vi "Main Monitor Loop.vi"(8 "error in (no error)":errorcluster, 11 "main ref":T1) -> (0 "error out":errorcluster)   [LabVIEW 2025]
uses:
  controls/LAB-IQ UI Data.ctl
  Traction Loop/Traction Receipe Enum.ctl
  <vilib>/Utility/error.llb/Trim Whitespace One-Sided.vi
panel:
  out "TDMS CLOSE":bool
  out "tdms file out":refnum<k34>
  out "File Create Temp":bool
  out "error out 2":errorcluster
  out "Test Stop Temp":bool
  out "DepthZ":dbl
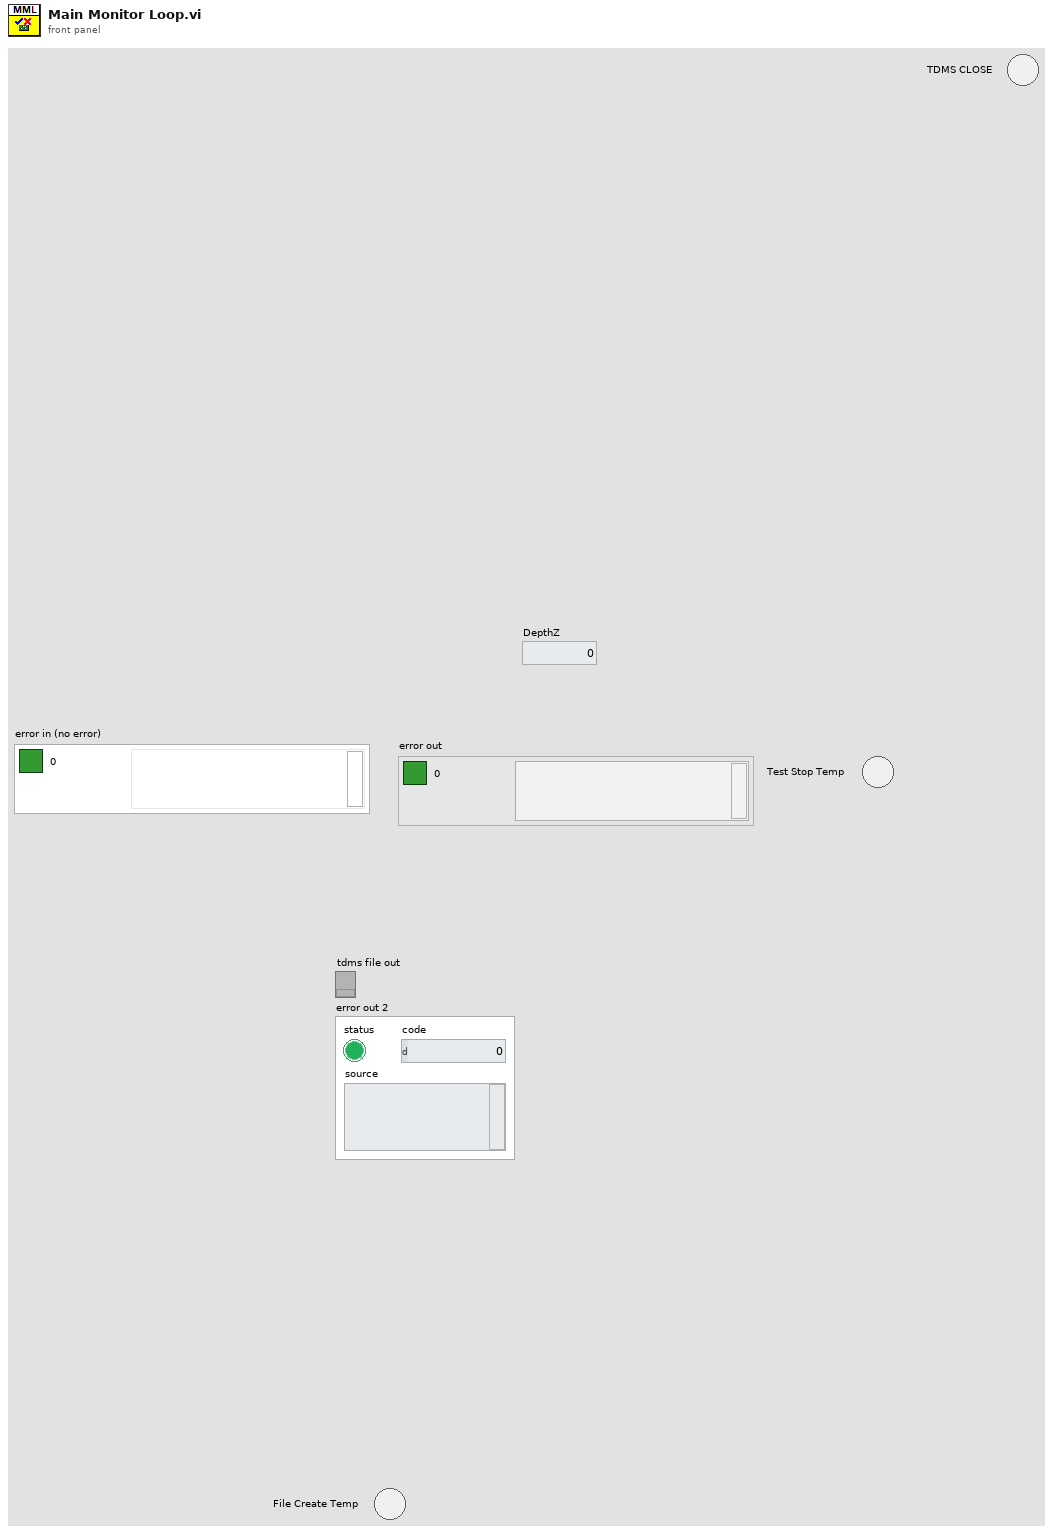
[diagram p1: front panel]
types:
  T1 = typedef "LAB-IQ UI Data.ctl" = cluster{"Main Home Screen":cluster{"GUI":refnum<vi>, "Platform Settings":refnum<vi>, "Configure":refnum<vi>, "Home":refnum<vi>, "EXIT":refnum<vi>, "service 2":refnum<vi>, "MainPage":refnum<vi>, "Analysis":refnum<vi>}, "Platform Settings":cluster{"mm/s  Surge":refnum<vi>, "Drive Error":refnum<vi>, "Disable Axis Jog Soft Limits":refnum<vi>, "mm/s  Sway":refnum<vi>, "Sway and Surge COM Status":refnum<vi>, "Heave COM Status":refnum<vi>, "Enable Platform":refnum<vi>, "Surge Forward Main":refnum<vi>, "Sway Right Main":refnum<vi>, "Sway Left Main":refnum<vi>, "Heave Down Main":refnum<vi>, "Heave Up main":refnum<vi>, "mm/s Heave":refnum<vi>, "mm/sec":refnum<vi>, "mm":refnum<vi>, "Surge Backward Main":refnum<vi>}, "Analysis Screen":cluster{"Analysis Home":refnum<vi>, "Surface Analysis":refnum<vi>, "Imaging":refnum<vi>, "Image Analysis":refnum<vi>, "Post Analysis":refnum<vi>}, "Config Screen":cluster{"Select Load Head":refnum<vi>, "Notes :":refnum<vi>, "FILE":refnum<vi>, "Sample ID :":refnum<vi>, "Operator ID :":refnum<vi>, "Operator Name :":refnum<vi>, "Auto":refnum<vi>}, "Motion Module":cluster{"zNL":refnum<vi>, "NL disp":refnum<vi>, "Rotary Tab":refnum<vi>, "Motion Direction:  3":refnum<vi>, "E.Velocity 2":refnum<vi>, "e.v/ssr 2":refnum<vi>, "Enter Fixed E.Velocity 2":refnum<vi>, "Enter Final SRR 2":refnum<vi>, "Enter initial SRR 2":refnum<vi>, "Enter Fixed SRR 2":refnum<vi>, "Enter the Final E.Velocity (m/s) 2":refnum<vi>, "Enter initial E.Velocity (m/s) 2":refnum<vi>, "Final Speed (RPM) 3":refnum<vi>, "Initial Speed (RPM) 2":refnum<vi>, "Enter the Final Velocity (m/s) 3":refnum<vi>, "Enter initial Velocity (m/s)  3":refnum<vi>, "Ramp Up 2":refnum<vi>, "TEST SELECTION":refnum<vi>, "SPEED SELECTION : ":refnum<vi>, "Angular Oscillation Set":refnum<vi>, "Traction":refnum<vi>, "Step Speed":refnum<vi>, "StepTable For Load-Speed":refnum<vi>, "StepTable For Speed":refnum<vi>, "Surge Forward MM":refnum<vi>, "Surge Backward MM":refnum<vi>, "M3 Image":refnum<vi>, "String 39":refnum<vi>, "Sway Left MM":refnum<vi>, "Sway Right MM":refnum<vi>, "Disable Axis Jog Soft Limits":refnum<vi>, "mm":refnum<vi>, "Heave Down MM":refnum<vi>, "Heave Up MM":refnum<vi>, "Wear Track Diameter (mm)":refnum<vi>, "Set WTD":refnum<vi>, "HomeScratch":refnum<vi>, "HomeRot":refnum<vi>, "PlaceModule":refnum<vi>, "Enter the Angle (Deg)":refnum<vi>, "Enter the Frequency (Hz)":refnum<vi>, "Motion Mode:":refnum<vi>, "LR Sway":refnum<vi>, "Rot Hor":refnum<vi>, "Scratch":refnum<vi>, "LR Cam":refnum<vi>, "MMBack":refnum<vi>, "MMNext":refnum<vi>, "Rot Ver":refnum<vi>, "Rotary Module Selection":refnum<vi>, "calculate rotary":refnum<vi>, "SPEED SELECTION : rotary":refnum<vi>, "Import 2":refnum<vi>, "Save 2":refnum<vi>, "File Path :  2":refnum<vi>, "String 45":refnum<vi>, "StepTable For Speed 3":refnum<vi>, "Enter the Speed(mm/sec)":refnum<vi>, "Enter the Speed(RPM)":refnum<vi>, "Enter Scratch Speed (mm/s):":refnum<vi>, "SwaySpeed Set":refnum<vi>, "Scartch Offset":refnum<vi>, "Motion type:":refnum<vi>, "HomeScratch 2":refnum<vi>, "Enter Scratch length (mm):":refnum<vi>, "Wear Track Diameter":refnum<vi>, "Rotary Speed Exced":refnum<vi>, "Scratch Mode":refnum<vi>, "No of Scratch":refnum<vi>}, "Environmental control":cluster{"Humidity  Status  3":refnum<vi>, "Low Temp  Status  2":refnum<vi>, "TK4 status 2":refnum<vi>, "Stage Temperature":refnum<vi>, "Sample Temperature":refnum<vi>, "Humidity (Amb)":refnum<vi>, "Clear List":refnum<vi>, "Add to list":refnum<vi>, "Wear":refnum<vi>, "Vibration":refnum<vi>, "Humidity (Chamber)":refnum<vi>, "Temperature (Chamber)":refnum<vi>, "ECR ":refnum<vi>, "Temperature (Amb)":refnum<vi>, "Microphone":refnum<vi>, "Acoustic Emission 3":refnum<vi>, "SNext":refnum<vi>, "APBack":refnum<vi>, "Enter the Temperature (°C):":refnum<vi>, "Enter the Stage \nTemperature (°C):":refnum<vi>, "Enter the Humidity (%Rh):":refnum<vi>, "Low Temp":refnum<vi>, "High Temp":refnum<vi>, "Humidity":refnum<vi>, "Sensors Picked":refnum<vi>}, "About Screen":cluster{"Password":refnum<vi>, "Home Service":refnum<vi>, "Advanced Setting":refnum<vi>, "About Tab":refnum<vi>, "ECR Port:":refnum<vi>, "Ramp Port:":refnum<vi>, "Installation/Replacement completed":refnum<vi>, "Loahead":refnum<vi>, "Heave and Surge COM Port:":refnum<vi>, "Sway COM Port:":refnum<vi>, "Temp Modbus:":refnum<vi>, "Humidity Port:":refnum<vi>, "Edit Gain Constants":refnum<vi>, "Save Gain Constants":refnum<vi>}, "Main Screen":cluster{"Main Screen Tab":refnum<vi>, "Angle and Frequency":refnum<vi>, "Stroke (mm)":refnum<vi>, "Angle (Deg)":refnum<vi>, "Main Speed Tab":refnum<vi>, "MTM MOTOR DISPLAY":refnum<vi>, "Disc Speed (m/sec)":refnum<vi>, "Ball Speed (m/sec)":refnum<vi>, "Disc Speed (RPM)":refnum<vi>, "Ball Speed (RPM)":refnum<vi>, "SPEED TAB":refnum<vi>, "Speed (m/sec)":refnum<vi>, "Set Speed (m/sec)":refnum<vi>, "Speed (RPM)":refnum<vi>, "Set Speed":refnum<vi>, "Time Tab":refnum<vi>, "Time ( HH:MM:SS ) 2":refnum<vi>, "Test Duration":refnum<vi>, "Test Duration 4":refnum<vi>, "TEST CYCLE":refnum<vi>, "TOTAL CYCLES":refnum<vi>, "Set Load (N)":refnum<vi>, "Temp Tabs":refnum<vi>, "Heater":refnum<vi>, "TK4 status":refnum<vi>, "ChamberTemp":refnum<vi>, "SetTmp":refnum<vi>, "Controller  Status":refnum<vi>, "ChamberTemp 2":refnum<vi>, "SetTmp 2":refnum<vi>, "Controller  Status 2":refnum<vi>, "ChamberTemp 3":refnum<vi>, "SetTmp 3":refnum<vi>, "Cooling":refnum<vi>, "Load Communication":refnum<vi>, "Ambient \nTemperature":refnum<vi>, "HumCOMStatus":refnum<vi>, "Ambient\n Humidity":refnum<vi>, "Freq (Hz)":refnum<vi>, "Load En":refnum<vi>, "NLt":refnum<vi>, "zNL 2":refnum<vi>, "Humidity On":refnum<vi>, "humidity disp":refnum<vi>, "Set Humidity":refnum<vi>, "NL disp 2":refnum<vi>, "Humidity On 2":refnum<vi>, "humidity disp 2":refnum<vi>, "Set Humidity 2":refnum<vi>, "NL disp 3":refnum<vi>, "AppLoadSeq scratch":refnum<vi>, "Stop Scratch":refnum<vi>, "ClrLog":refnum<vi>, "Trip Log":refnum<vi>, "STOP":refnum<vi>, "Start Test":refnum<vi>, "Test status":refnum<vi>, "AR Led":refnum<vi>, "Data":refnum<vi>, "Health":refnum<vi>, "Sway COM Status":refnum<vi>, "Heave COM Status":refnum<vi>, "Grp Tab":refnum<vi>, "Sub Graph":refnum<vi>, "SD (mm)":refnum<vi>, "Siliding distance Reset Graph":refnum<vi>, "SDGp":refnum<vi>, "Humidity Reset Graph":refnum<vi>, "HumrGp":refnum<vi>, "Acoustic Emission (mV)":refnum<vi>, "Aqucostic Reset Graph":refnum<vi>, "gACQUOS":refnum<vi>, "ECR RESET":refnum<vi>, "ECR":refnum<vi>, "Temperature Reset":refnum<vi>, "Acoustic Emission (mV) 2":refnum<vi>, "Aqucostic Reset Graph 2":refnum<vi>, "gACQUOS 2":refnum<vi>, "ECR RESET 2":refnum<vi>, "ECR 2":refnum<vi>, "Temperature Reset 2":refnum<vi>, "Temperature (deg c)":refnum<vi>, "Speed Reset Graph":refnum<vi>, "Speed Tab":refnum<vi>, "MTM DISC  SPEED":refnum<vi>, "MTM BALL SPEED":refnum<vi>, "speed mm/sec":refnum<vi>, "Hymidity":refnum<vi>, "Humidity Disable trip":refnum<vi>, "CoF Trip  2":refnum<vi>, "Depth Trip":refnum<vi>, "Weart Deapth":refnum<vi>, "Depth Reset Graph":refnum<vi>, "Weart":refnum<vi>, "Depthz":refnum<vi>, "Depth (µm)":refnum<vi>, "WearGp":refnum<vi>, "NL Trip 2":refnum<vi>, "Load pid":refnum<vi>, "Load Disable Trip":refnum<vi>, "Load Reset Graph":refnum<vi>, "NL Display 4":refnum<vi>, "Main Chart 3":refnum<vi>, "BACK":refnum<vi>, "Depth Trip 2":refnum<vi>, "COF TRIP ":refnum<vi>, "Friction Force (N)":refnum<vi>, "FF Reset Graph":refnum<vi>, "FF Disable Trip":refnum<vi>, "FF TRIP":refnum<vi>, "COF Disable Trip":refnum<vi>, "COF Reset Graph":refnum<vi>, "Start Test Temp":refnum<vi>, "zFF":refnum<vi>, "Friction Force (N) Graph":refnum<vi>, "Coefficient of Friction":refnum<vi>, "Scratch Start Test":refnum<vi>, "FF Tab":refnum<vi>, "Cyclic Friction Force (N)":refnum<vi>, "CZ FF":refnum<vi>, "Cyclic Friction Force (N) Graph":refnum<vi>, "Cyclic Coefficient of Friction":refnum<vi>, "Cyclic FF TRIP":refnum<vi>, "Cyclic FF Disable Trip":refnum<vi>, "cyclic COF Disable Trip":refnum<vi>, "cyclic COF TRIP":refnum<vi>, "cyclic COF Reset Graph":refnum<vi>, "Cyclic FF Reset Graph":refnum<vi>, "Test Trip":refnum<vi>, "Multi Scratch Pass":refnum<vi>, "Scratch Start Recording":refnum<vi>}, "Loading":cluster{"Indentation":refnum<vi>, "Reference Sample":refnum<vi>, "Load Cell Communication Slide":refnum<vi>, "com 3":refnum<vi>, "com":refnum<vi>, "DecaForce COM Status":refnum<vi>, "Update":refnum<vi>, "Clear 3":refnum<vi>, "seq":refnum<vi>, "Stribeck table":refnum<vi>, "Stribeck Table  For loading":refnum<vi>, "Loading Mode":refnum<vi>, "Enter the Final Load (N)":refnum<vi>, "Enter the CoF Trip":refnum<vi>, "Enter the Friction Force Trip":refnum<vi>, "Enter the Normal load Trip":refnum<vi>, "Enter the Load  (N)":refnum<vi>, "KiloForce":refnum<vi>, "DecaForce ":refnum<vi>, "MicroForce":refnum<vi>, "LHBack":refnum<vi>, "LHNext":refnum<vi>, "Enter the Loading Rate (N/min)":refnum<vi>, "Message":refnum<vi>, "Warning 2":refnum<vi>, "SSP 0.75":refnum<vi>, "SSP 0.5":refnum<vi>, "SSP 0.3":refnum<vi>, "Warning":refnum<vi>, "gui GIF":refnum<vi>, "Communication is established":refnum<vi>, "AppLoad 4":refnum<vi>, "Multipoint":refnum<vi>, "Load Selection":refnum<vi>}, "PID":cluster{"Ramp":refnum<vi>, "Vertical load (N)":refnum<vi>, "apply load":refnum<vi>, "apply load 2":refnum<vi>, "Enter ByPass Load":refnum<vi>, "Bypass Load":refnum<vi>, "gFF Rot":refnum<vi>}, "Config Parameters":cluster{"Tab Control 3":refnum<vi>, "Tab Control 19":refnum<vi>, "SAMPLES":refnum<vi>, "Re-initilaize":refnum<vi>, "Filter ON/OFF":refnum<vi>, "TracHomeSurgeOffsetCounts 10MM":refnum<vi>, "TracHomeSwayOffsetCounts 10MM":refnum<vi>, "Acoustic Emission:":refnum<vi>, "Apply Filter (FF)":refnum<vi>, "Filter% 2":refnum<vi>, "Apply Filter (Load)":refnum<vi>, "Filter% ":refnum<vi>, "Sway distance (mm)":refnum<vi>, "Surge distance (mm)":refnum<vi>, "DataSavingLoopDelay(ms)":refnum<vi>, "SAVE 2":refnum<vi>, "Enter Distance":refnum<vi>, "Sway Counts:":refnum<vi>, "Distance (mm): 3":refnum<vi>, "Surge Counts:":refnum<vi>, "Distance (mm): 2":refnum<vi>, "Distance (mm):":refnum<vi>, "Heave Counts:":refnum<vi>, "LRMHomeSurgeOffsetCounts":refnum<vi>, "LRMHomeSwayOffsetCounts":refnum<vi>, "TracHomeSurgeOffsetCounts 20MM":refnum<vi>, "TracHomeSwayOffsetCounts 20MM":refnum<vi>, "RotHomeSwayOffsetCounts":refnum<vi>, "RotHomeSurgeOffsetCounts":refnum<vi>, "Heave distance":refnum<vi>, "Zmm":refnum<vi>, "Heave Pulses/mm":refnum<vi>, "Surge Pulses/mm":refnum<vi>, "Sway Pulses/mm":refnum<vi>, "Heave Pitch":refnum<vi>, "Surge Pitch":refnum<vi>, "Sway Pitch":refnum<vi>, "Heave PPR":refnum<vi>, "Surge PPR":refnum<vi>, "Sway PPR":refnum<vi>, "Tab Control 5":refnum<vi>, "Tab Control 14":refnum<vi>, "Tab Control 26":refnum<vi>, "AE":refnum<vi>, "Heave Loop Delay":refnum<vi>, "Heave PID Speed":refnum<vi>, "Surge Jog Speed":refnum<vi>, "Heave Jog Speed":refnum<vi>, "Sway Loop Delay":refnum<vi>, "Sway PID Speed":refnum<vi>, "Sway Jog Speed":refnum<vi>, "DEPTH TRIP VALUE":refnum<vi>, "LOAD TRIP VALUE":refnum<vi>, "DEPTH TRIP   ENABLE":refnum<vi>, "LOAD TRIP  ENABLE":refnum<vi>, "CYCLIC FF TRIP VALUE":refnum<vi>, "FF TRIP VALUE":refnum<vi>, "CYCLIC CoF TRIP VALUE":refnum<vi>, "COF TRIP VALUE":refnum<vi>, "CYCLIC COF TRIP  ENABLE":refnum<vi>, "CYCLIC FF TRIP  ENABLE":refnum<vi>, "FF TRIP  ENABLE":refnum<vi>, "COF TRIP  ENABLE":refnum<vi>, "JOG TRIP LOAD VALUE (N)":refnum<vi>, "Rotary Vertical":refnum<vi>, "Traction":refnum<vi>, "Scratch":refnum<vi>, "LRM CAM":refnum<vi>, "Sway LRM":refnum<vi>, "Rotary Horizontal":refnum<vi>}, "Loading Com Port":cluster{"ClearAll":refnum<vi>, "Mz(Nm)":refnum<vi>, "My(Nm)":refnum<vi>, "Mx(Nm)":refnum<vi>, "Save Dwell":refnum<vi>, "Acq Delay (ms)":refnum<vi>, "Burst Delay (ms)":refnum<vi>, "model":refnum<vi>, "SN":refnum<vi>, "FFx(N)":refnum<vi>, "Sensor IP":refnum<vi>, "Port":refnum<vi>, "FFy(N)":refnum<vi>, "Load(N)":refnum<vi>, "delete Handle":refnum<vi>, "Create Handle":refnum<vi>, "ft_data":refnum<vi>, "ft_range":refnum<vi>, "ft_data 2":refnum<vi>, "stop 6":refnum<vi>, "running_flag":refnum<vi>, "ft_udp_handle":refnum<vi>, "get-data-return":refnum<vi>, "get-range-return":refnum<vi>, "zero-return":refnum<vi>, "filter-return":refnum<vi>, "initial-return":refnum<vi>, "deleteHandle-result":refnum<vi>, "Load Cell Temp":refnum<vi>, "Load Cell":refnum<vi>, "ZeroAll":refnum<vi>, "FORCE (N)":refnum<vi>, "TORQUE (N-m)":refnum<vi>, "Load Cell Link":refnum<vi>}, "Heave AND Surge":cluster{"SURGE POSE":refnum<vi>, "error out Read":refnum<vi>, "HEAVE POSE":refnum<vi>, "State":refnum<vi>, "Homed":refnum<vi>, "Sequence ID":refnum<vi>, "error out Write":refnum<vi>, "faultCode":refnum<vi>, "Ack ID":refnum<vi>, "SPEED":refnum<vi>, "Distance":refnum<vi>, "Mode Command":refnum<vi>, "Heave and Surge Read":refnum<vi>, "Read Heave Temp":refnum<vi>, "Spare 15":refnum<vi>, "Spare 14":refnum<vi>, "Spare 13":refnum<vi>, "Spare 12":refnum<vi>, "Spare 11":refnum<vi>, "Spare 10":refnum<vi>, "Spare 9":refnum<vi>, "Spare 8":refnum<vi>, "Spare 7":refnum<vi>, "Spare 4":refnum<vi>, "Spare 3":refnum<vi>, "Spare 2":refnum<vi>, "Humidity":refnum<vi>, "Temp":refnum<vi>, "Node Id":refnum<vi>, "Spare 1":refnum<vi>, "SPARE 4":refnum<vi>, "SPARE 3":refnum<vi>, "SPARE 2":refnum<vi>, "SPARE 1":refnum<vi>, "fwMajor":refnum<vi>, "fwMinor":refnum<vi>, "Manual Write":refnum<vi>, "Heave and Surge Write":refnum<vi>, "SPARE 5":refnum<vi>, "Reserved ":refnum<vi>, "SPARE 8":refnum<vi>, "SPARE 6":refnum<vi>, "SPARE 7":refnum<vi>, "SPARE 17":refnum<vi>, "SPARE 16":refnum<vi>, "SPARE 15":refnum<vi>, "SPARE 14":refnum<vi>, "SPARE 13":refnum<vi>, "SPARE 12":refnum<vi>, "SPARE 11":refnum<vi>, "SPARE 10":refnum<vi>, "SPARE 9":refnum<vi>, "System UPTIME":refnum<vi>, "Missed Packets":refnum<vi>, "faultCode Surge Right":refnum<vi>, "faultCode Surge Left":refnum<vi>, "faultCode Heave":refnum<vi>, "UPLINK HEAVE":refnum<vi>, "DOWNLINK HEAVE":refnum<vi>}, "New PID LOGIC":cluster{"Fine Tune Zone":refnum<vi>, "PID SDelay":refnum<vi>, "Max_pos_limit":refnum<vi>, "Min_pos_limit":refnum<vi>, "i_limit":refnum<vi>, "pct_scale":refnum<vi>, "Deadband":refnum<vi>, "Kd":refnum<vi>, "Ki":refnum<vi>, "Kp":refnum<vi>, "Current Position":refnum<vi>, "Set Load":refnum<vi>, "Current Load":refnum<vi>, "Pulse delta":refnum<vi>, "Init Step":refnum<vi>, "Max Step Linit":refnum<vi>, "min_deadband_floor":refnum<vi>, "dynamic_spindle_noise_scalar":refnum<vi>, "min_finetune_floor":refnum<vi>, "filter_alpha":refnum<vi>, "PID":refnum<vi>}, "SWAY ":cluster{"fwMajor":refnum<vi>, "Homed":refnum<vi>, "Rotary POSE":refnum<vi>, "State":refnum<vi>, "SWAY POSE":refnum<vi>, "Ack ID":refnum<vi>, "faultCode":refnum<vi>, "Node Id":refnum<vi>, "fwMinor":refnum<vi>, "Spare 6":refnum<vi>, "Spare 5":refnum<vi>, "Spare 4":refnum<vi>, "Spare 3":refnum<vi>, "Spare 2":refnum<vi>, "Spare 1":refnum<vi>, "Spare 7":refnum<vi>, "SPARE  5":refnum<vi>, "error out Write  SWAY ":refnum<vi>, "error out Read SWAY ":refnum<vi>, "Manual Write SWAY ":refnum<vi>, "SWAY WRITE":refnum<vi>, "SPARE  4":refnum<vi>, "SPARE  3":refnum<vi>, "SPARE 2":refnum<vi>, "SPARE 1":refnum<vi>, "Spare 15":refnum<vi>, "Spare 14":refnum<vi>, "Spare 13":refnum<vi>, "Spare 12":refnum<vi>, "Spare 11":refnum<vi>, "Spare 9":refnum<vi>, "Spare 8":refnum<vi>, "SPEED":refnum<vi>, "Distance":refnum<vi>, "Mode Command":refnum<vi>, "Sequence ID":refnum<vi>, "SWAY READ":refnum<vi>, "Spare 10":refnum<vi>, "Read SWAY Temp":refnum<vi>, "faultCode Sway ":refnum<vi>, "Missed Packets":refnum<vi>, "System UPTIME sway":refnum<vi>, "SPARE 6":refnum<vi>, "SPARE 7":refnum<vi>, "SPARE 9":refnum<vi>, "SPARE 11":refnum<vi>, "SPARE 10":refnum<vi>, "SPARE 8":refnum<vi>, "SPARE 13":refnum<vi>, "SPARE 12":refnum<vi>, "SPARE 17":refnum<vi>, "SPARE 16":refnum<vi>, "SPARE 15":refnum<vi>, "SPARE 14":refnum<vi>, "Reserved":refnum<vi>, "faultCode Rotary":refnum<vi>, "UPLINK SWAY":refnum<vi>, "DOWNLINK SWAY":refnum<vi>}, "Analysis Screen":cluster{"Analysis Home":refnum<vi>, "Refresh 2":refnum<vi>, "MEAN 4":refnum<vi>, "SD 4":refnum<vi>, "VARIANCE 4":refnum<vi>, "MEAN  3":refnum<vi>, "SD  3":refnum<vi>, "VARIANCE  3":refnum<vi>, "MEAN 2":refnum<vi>, "SD  2":refnum<vi>, "VARIANCE 2":refnum<vi>, "MEAN":refnum<vi>, "SD":refnum<vi>, "VARIANCE":refnum<vi>, "File 4 Discription":refnum<vi>, "OPEN 4":refnum<vi>, "File Name 4":refnum<vi>, "OPEN 3":refnum<vi>, "File 3 Discription":refnum<vi>, "File Name 3":refnum<vi>, "Y-AXIS":refnum<vi>, "X-AXIS":refnum<vi>, "XY Graph":refnum<vi>, "File Name 2":refnum<vi>, "File Name 1":refnum<vi>, "OPEN 2":refnum<vi>, "OPEN 1":refnum<vi>, "File 1 Discription ":refnum<vi>, "File 2 Discription":refnum<vi>, "Export":refnum<vi>, "File Format":refnum<vi>}, "Traction":cluster{"faultCode Traction 2":refnum<vi>, "faultCode Traction 1":refnum<vi>, "Missed Packets":refnum<vi>, "System UPTIME Traction":refnum<vi>, "SPARE 17":refnum<vi>, "SPARE 16":refnum<vi>, "SPARE 15":refnum<vi>, "SPARE 14":refnum<vi>, "SPARE 13":refnum<vi>, "SPARE 12":refnum<vi>, "SPARE 11":refnum<vi>, "SPARE 10":refnum<vi>, "SPARE 9":refnum<vi>, "SPARE 8":refnum<vi>, "SPARE 7":refnum<vi>, "SPARE 6":refnum<vi>, "Reserved":refnum<vi>, "SPARE  5":refnum<vi>, "Manual Write TRACTION":refnum<vi>, "TRACTION WRITE":refnum<vi>, "SPARE  4":refnum<vi>, "SPARE  3":refnum<vi>, "SPARE 2":refnum<vi>, "SPARE 1":refnum<vi>, "Spare 7":refnum<vi>, "Spare 6":refnum<vi>, "Spare 5":refnum<vi>, "Spare 4":refnum<vi>, "Spare 2":refnum<vi>, "Spare 1":refnum<vi>, "Node Id":refnum<vi>, "Read TRACTION Temp":refnum<vi>, "fwMinor":refnum<vi>, "fwMajor":refnum<vi>, "faultCode":refnum<vi>, "TRACTION POSE":refnum<vi>, "TRACTION POSE 2":refnum<vi>, "Homed":refnum<vi>, "State":refnum<vi>, "Ack ID":refnum<vi>, "SPEED":refnum<vi>, "Distance":refnum<vi>, "Mode Command":refnum<vi>, "Sequence ID":refnum<vi>, "error out Read TRACTION":refnum<vi>, "error out Write  TRACTION":refnum<vi>, "TRACTION READ":refnum<vi>, "Spare 3":refnum<vi>, "Downlink traction":refnum<vi>, "Uplink Traction":refnum<vi>}, "Traction reciepe":cluster{"SRR Sweep Range (%) Stribeck":refnum<vi>, "Traction Receipe":refnum<vi>, "Total Execution Time":refnum<vi>, "Total Steps":refnum<vi>, "Duration / Step (s)  Stribeck":refnum<vi>, "STRIBECK Fixed SRR List (%)":refnum<vi>, "Duration / Step (s) Traction":refnum<vi>, "SRR Sweep Range (%) traction":refnum<vi>, "Rolling Speed (mm/s)":refnum<vi>, "Temperature Stages (°C)":refnum<vi>, "Ball Load (N)":refnum<vi>, "Lubricant Name":refnum<vi>, "Profile File Name":refnum<vi>, "SET entrainment Velocity":refnum<vi>, "Test Array Size":refnum<vi>, "SRR INDEX [ STRIBECK]":refnum<vi>, "Stribeck Size":refnum<vi>, "SET SRR":refnum<vi>, "ELAPSED TIMER ":refnum<vi>, "BALL SET RPM":refnum<vi>, "DISC SET RPM":refnum<vi>, "SET LOAD":refnum<vi>, "TEMPERATURE READ":refnum<vi>, "SET TEMPERATURE":refnum<vi>, "Traction Size":refnum<vi>, "DISC SPEED (rpm)":refnum<vi>, "BALL SPEED (rpm)":refnum<vi>, "BALL WEAR TRACK":refnum<vi>, "DISC WEARTRACK":refnum<vi>, "SRR INDEX [ TRACTION]":refnum<vi>, "Start Index Type":refnum<vi>, "Enum - Menu":refnum<vi>, "Ball (mm/sec)":refnum<vi>, "Disc (mm/sec)":refnum<vi>}, "Traction Control":cluster{"HomeTraction":refnum<vi>, "Demo Mode Display":refnum<vi>, "Traction Message":refnum<vi>, "Traction Step Update Details":refnum<vi>, "Main Tab sequence for selection":refnum<vi>, "Ramp Tab":refnum<vi>, "e.v/ssr":refnum<vi>, "Enter Fixed E.Velocity":refnum<vi>, "Enter Final SRR":refnum<vi>, "Enter initial SRR":refnum<vi>, "Enter Fixed SRR":refnum<vi>, "Enter the Final E.Velocity (m/s)":refnum<vi>, "Enter initial E.Velocity (m/s)":refnum<vi>, "Ball WTD":refnum<vi>, "E.Velocity":refnum<vi>, "Enter the Final Velocity (m/s)":refnum<vi>, "Enter initial Velocity (m/s)":refnum<vi>, "Ramp Up   Disc":refnum<vi>, "Initial DiscSpeed (RPM)":refnum<vi>, "Final Speed (RPM) Ball":refnum<vi>, "Final Speed (RPM)":refnum<vi>, "Initial Speed (RPM) Ball":refnum<vi>, "Enter the Final Velocity (m/s) Ball":refnum<vi>, "Enter initial Velocity (m/s) Ball":refnum<vi>, "Ramp Up":refnum<vi>, "ExceedBallSpeed step":refnum<vi>, "ExceedDiscSpeed":refnum<vi>, "BallSpeed Exceed Indication":refnum<vi>, "Apply":refnum<vi>, "SPEED SELECTION : MTM":refnum<vi>, "SPEED SELECTION : MTM 2":refnum<vi>, "TEST SELECTION (MTM)":refnum<vi>, "MTM Test Selection":refnum<vi>, "File Path Tab":refnum<vi>, "File Path String":refnum<vi>, "Save":refnum<vi>, "Save  2":refnum<vi>, "Import ":refnum<vi>, "File Path :":refnum<vi>, "Step Sequence Indication Tab":refnum<vi>, "Step Sequence Indication":refnum<vi>, "Calculate Step":refnum<vi>, "StepTable":refnum<vi>, "ExceedDiscSpeed  Cinstant Speed":refnum<vi>, "ExceedBallSpeed Constant":refnum<vi>, "TEST SELECTION (MTM) 2":refnum<vi>, "SPEED SELECTION : MTM 3":refnum<vi>, "MTM Test Selection 2":refnum<vi>, "Enter the Speed (m/sec): ":refnum<vi>, "Enter the Speed (m/sec):  2":refnum<vi>, "Enter the Speed (RPM):":refnum<vi>, "Lower Spped ":refnum<vi>, "Upper":refnum<vi>, "Enter the Speed (RPM):Ball":refnum<vi>, "Disc Motion Direction: ":refnum<vi>, "Ball Motion Direction :":refnum<vi>, "Motion Mode: ":refnum<vi>, "Wear Track Diameter (mm) ":refnum<vi>, "Disc Speed Indicator":refnum<vi>, "ExceedBallSpeed":refnum<vi>}, "Acquostic":cluster{"Last Config Rejected ":refnum<vi>, "rx command count":refnum<vi>, "Current Filter Id":refnum<vi>, "Isolated Gain":refnum<vi>, "DAQ Status":refnum<vi>, "error out":refnum<vi>, "error in (no error)":refnum<vi>, "Uplink Packet":refnum<vi>, "data out":refnum<vi>, "Downlink Packet":refnum<vi>, "Gains":refnum<vi>, "Manual Write Acquostic":refnum<vi>, "Acoustic Graphs":refnum<vi>}}
  T2 = enum32{"  Acquire  ", "Compare Files Rot", "About", "Service"}
  T3 = enum32{"Setup", "Load Head", "Motion Module", "Environment", "Begin"}
  T4 = enum16{"open", "open or create", "create or replace", "create", "open (read-only)"}
  T5 = cluster{"Ack ID":u16, "State":u8, "Homed":u8, "HEAVE POSE":sgl, "SURGE POSE":sgl, "faultCode":u16, "fwMajor":u8, "fwMinor":u8, "Node Id":u8, "Spare 1":u8, "Spare 2":u8, "Spare 3":u8, "Spare 4":u8, "Spare 5":u8, "Spare 6":u8, "Spare 7":u8, "System UPTIME":sgl, "Missed Packets":sgl, "faultCode Heave":u16, "faultCode Surge Left":u16, "faultCode Surge Right":u16}
  T6 = cluster{"Sequence ID":u32, "Timestamp":u32, "System Status":u32, "Peak Amplitude":sgl, "Amplitude dB_AE":sgl, "AE Ring-Down Counts":u32, "Signal Energy":sgl, "Spare 1":u32}
  T7 = cluster{"Ack ID ":u16, "State":u8, "Homed":u8, "SWAY POSE ":sgl, "Rotary POSE ":sgl, "faultCode":u16, "fwMajor":u8, "fwMinor":u8, "Node Id":u8, "Spare 1":u8, "Spare 2":u8, "Spare 3":u8, "Spare 4":u8, "Spare 5":u8, "Spare 6":u8, "Spare 7":u8, "System UPTIME ":sgl, "Missed Packets ":sgl, "faultCode Sway":u16, "faultCode Rotary":u16}
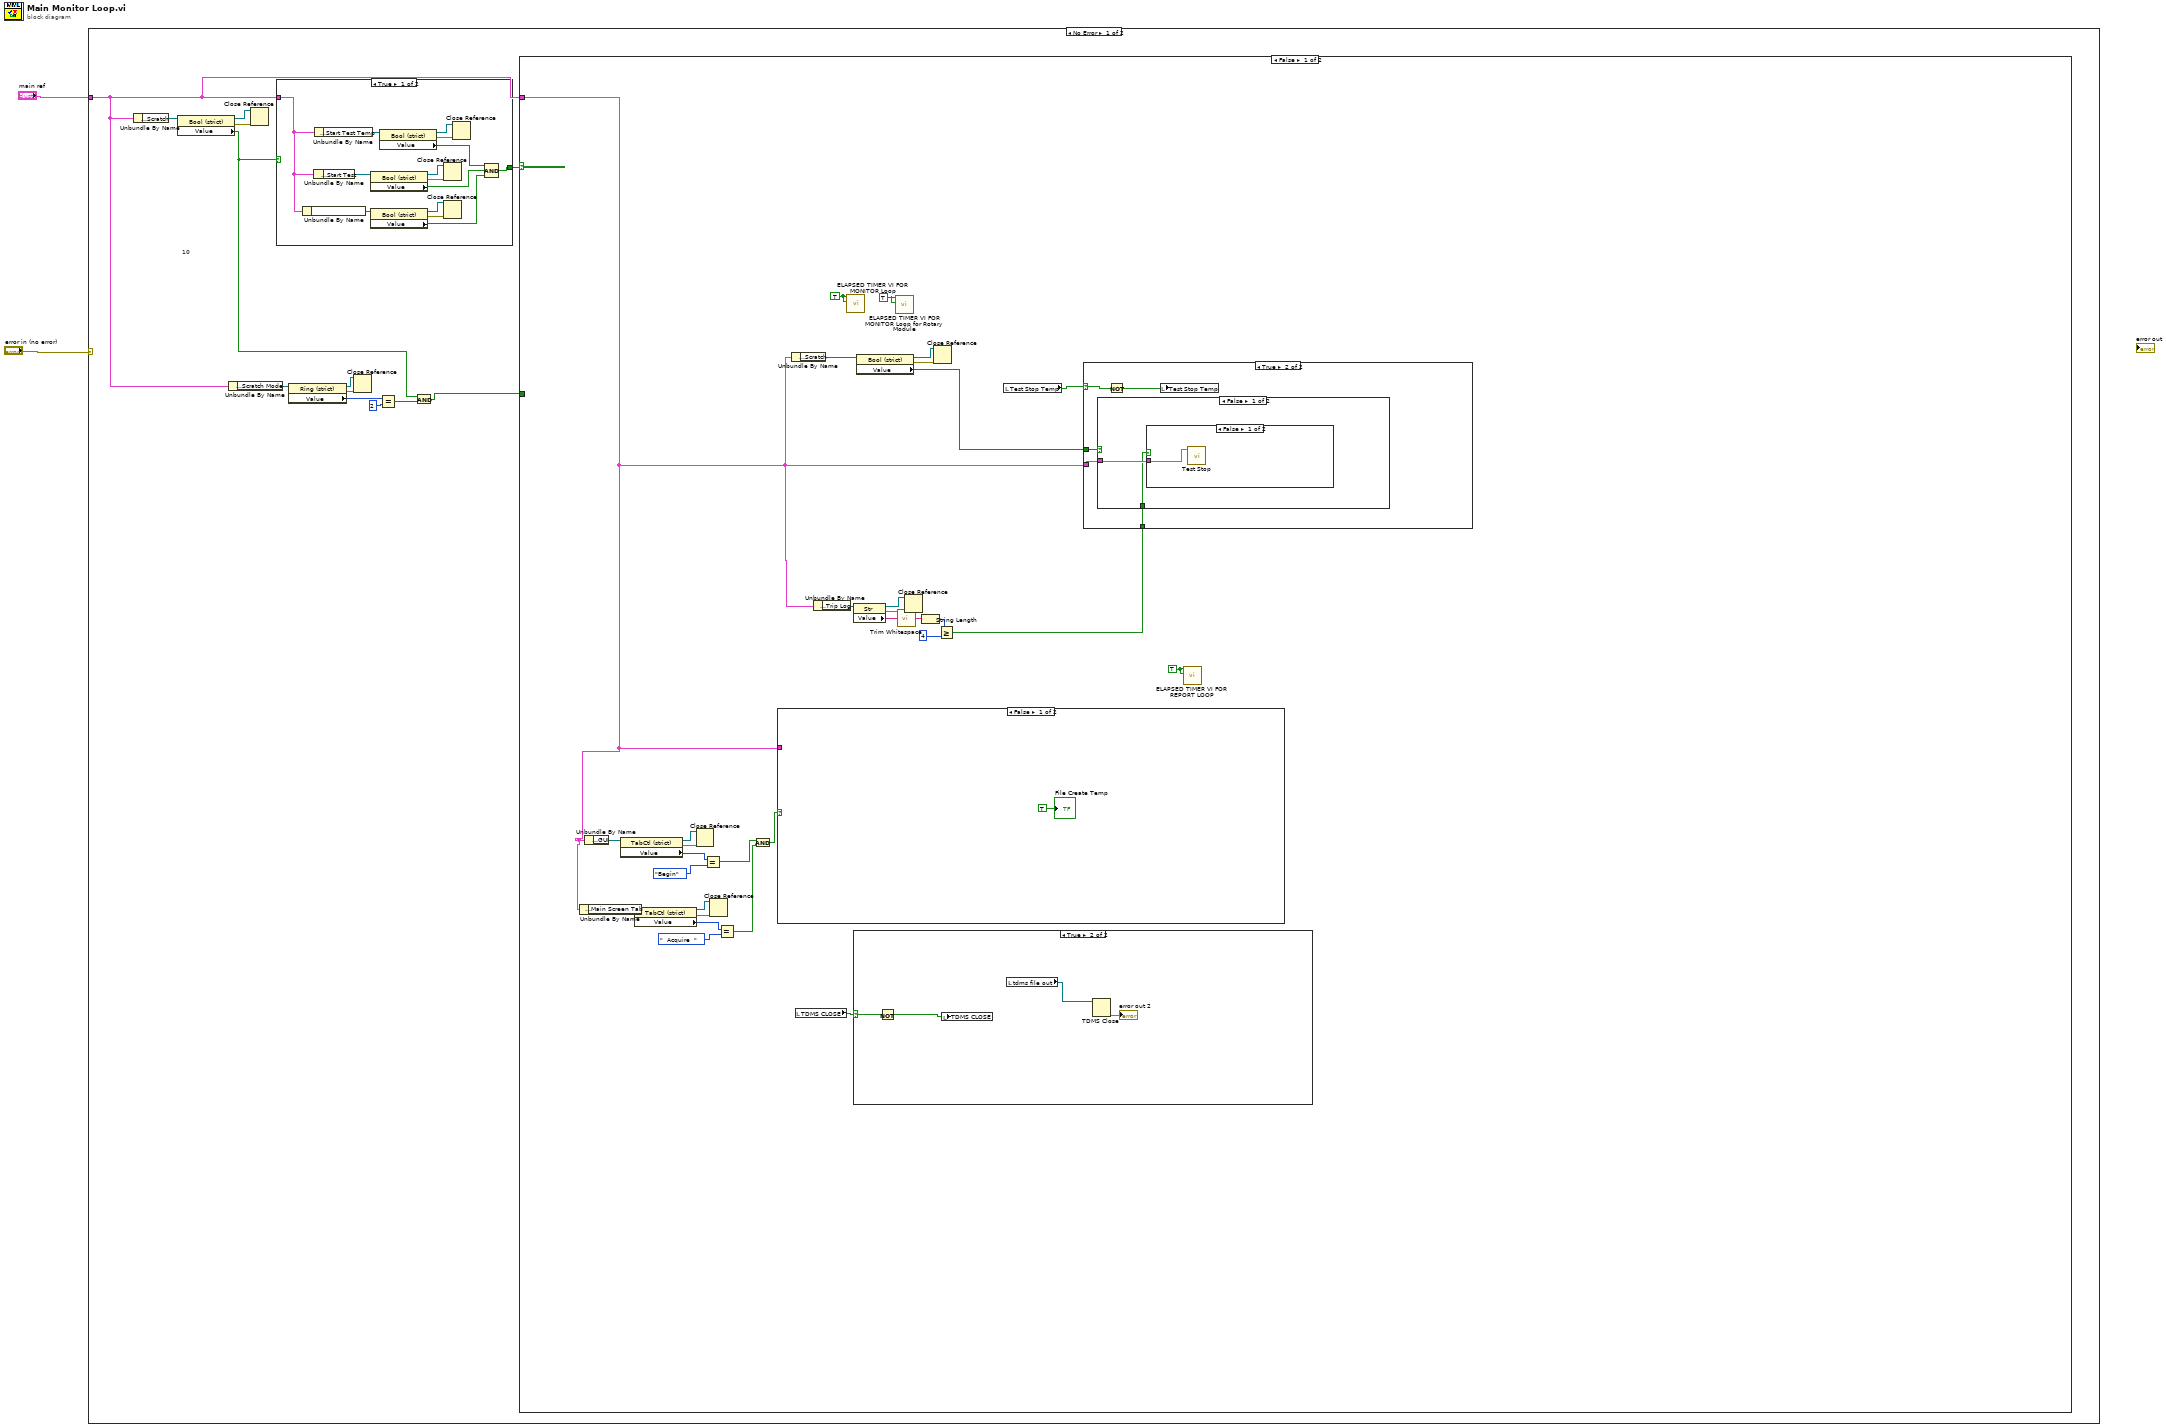
[diagram p0: block diagram]
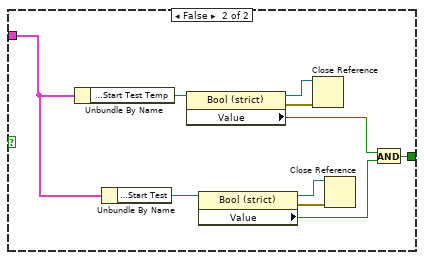
[diagram p2: hidden frame]
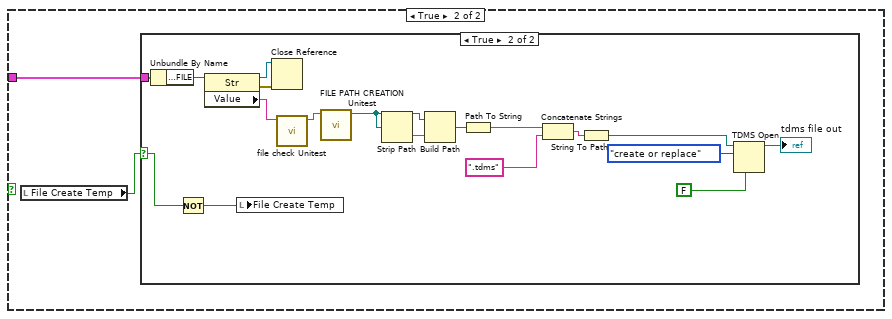
[diagram p4: hidden frame]
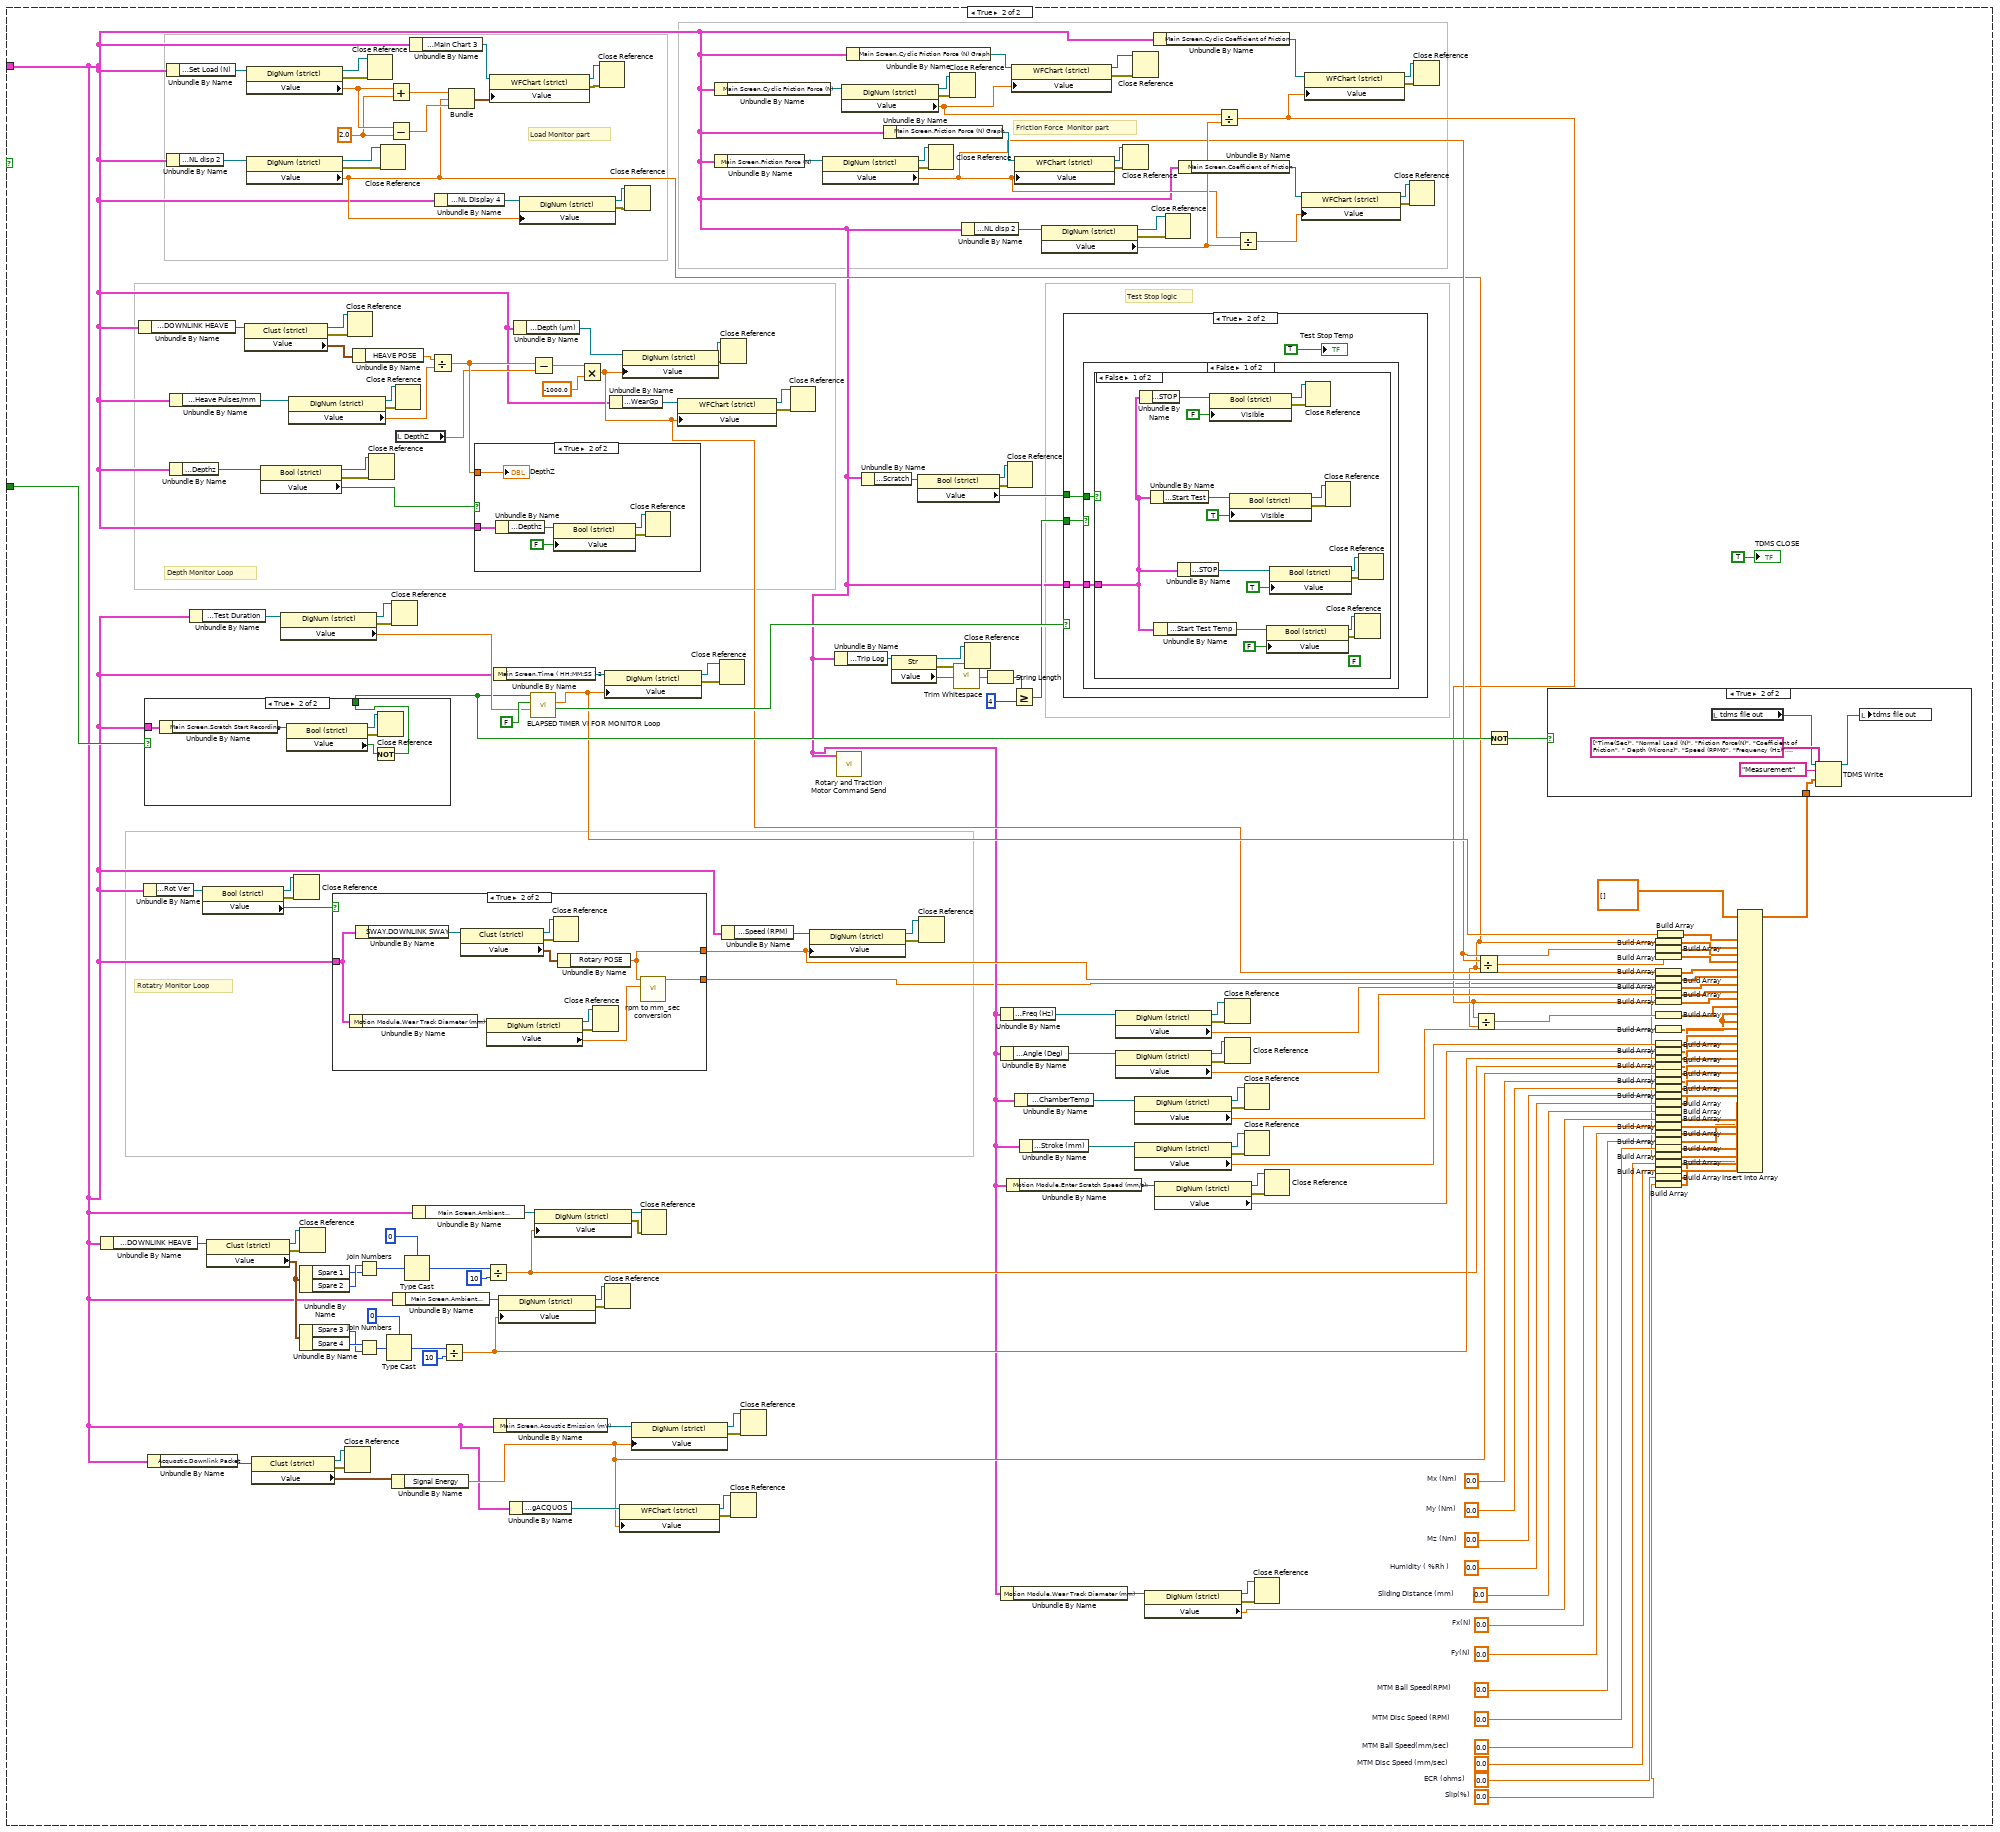
[diagram p9: hidden frame]
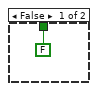
[diagram p11: hidden frame]
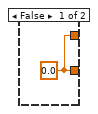
[diagram p12: hidden frame]
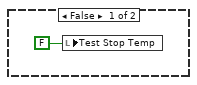
[diagram p13: hidden frame]
diagram:
  n1 = case shown="No Error" "error in (no error)" {
    tunnel: "main ref" -> [w4 _]
    frame No Error {
      # "10"
      n2 = Unbundle By Name(w4) -> ("Motion Module.Scratch"=w13:refnum<vi>)
      n3 = property class="Bool (strict)"(reference=w13) -> (reference out=w14:refnum<vi>, error out=w12:errorcluster, "Value"=w5:bool)  [unwired: 1 in]
      n4 = Unbundle By Name(w4) -> ("Motion Module.Scratch Mode"=w7:refnum<vi>)
      n5 = Close Reference(reference=w14, error in (no error)=w12) -> ()  [unwired: 1 out]
      n6 = case shown="True" w5 {
        tunnel: w4 -> [w17 w33]
        tunnel: [w21 w31] -> w15
        frame True {
          n7 = Unbundle By Name(w17) -> ("Main Screen.Scratch Start Test"=w19:refnum<vi>)
          n8 = Unbundle By Name(w17) -> ("Main Screen.Start Test"=w25:refnum<vi>)
          n9 = Unbundle By Name(w17) -> ("Main Screen.Start Test Temp"=w28:refnum<vi>)
          n10 = property class="Bool (strict)"(reference=w25) -> (reference out=w24:refnum<vi>, error out=w26:errorcluster, "Value"=w22:bool)  [unwired: 1 in]
          n11 = property class="Bool (strict)"(reference=w19) -> (reference out=w20:refnum<vi>, error out=w18:errorcluster, "Value"=w16:bool)  [unwired: 1 in]
          n12 = property class="Bool (strict)"(reference=w28) -> (reference out=w29:refnum<vi>, error out=w27:errorcluster, "Value"=w23:bool)  [unwired: 1 in]
          n13 = Close Reference(reference=w24, error in (no error)=w26) -> ()  [unwired: 1 out]
          n14 = Close Reference(reference=w20, error in (no error)=w18) -> ()  [unwired: 1 out]
          n15 = Close Reference(reference=w29, error in (no error)=w27) -> ()  [unwired: 1 out]
          n16 = Compound Arithmetic op=AND(w23, w22, w16) -> (w21:bool)
        }
        frame False {
          n17 = Unbundle By Name(w33) -> ("Main Screen.Start Test Temp"=w38:refnum<vi>)
          n18 = Unbundle By Name(w33) -> ("Main Screen.Start Test"=w35:refnum<vi>)
          n19 = property class="Bool (strict)"(reference=w38) -> (reference out=w39:refnum<vi>, error out=w37:errorcluster, "Value"=w32:bool)  [unwired: 1 in]
          n20 = property class="Bool (strict)"(reference=w35) -> (reference out=w34:refnum<vi>, error out=w36:errorcluster, "Value"=w30:bool)  [unwired: 1 in]
          n21 = Close Reference(reference=w39, error in (no error)=w37) -> ()  [unwired: 1 out]
          n22 = Close Reference(reference=w34, error in (no error)=w36) -> ()  [unwired: 1 out]
          n23 = And(x=w32, y=w30) -> (x .and. y?=w31:bool)
        }
      }
      n24 = property class="Ring (strict)"(reference=w7) -> (reference out=w6:refnum<vi>, error out=w8:errorcluster, "Value"=w9:u16)  [unwired: 1 in]
      n25 = Close Reference(reference=w6, error in (no error)=w8) -> ()  [unwired: 1 out]
      n26 = Equal?(x=w9, y=u16 2) -> (x = y?=w11:bool)
      n27 = Compound Arithmetic op=AND(w5, w11) -> (w3:bool)
      n28 = case shown="False" w15 {
        tunnel: w4 -> [w40 w114]
        tunnel: w3 -> [_ w190]
        frame False {
          w41 = TRUE ("PAUSE")
          w64 = TRUE ("PAUSE")
          w70 = TRUE ("PAUSE")
          n29 = Unbundle By Name(w40) -> ("Main Screen.Main Screen Tab"=w49:refnum<vi>)
          n30 = Unbundle By Name(w40) -> ("Main Home Screen.GUI"=w43:refnum<vi>)
          n31 = property class="TabCtl (strict)"(reference=w43) -> (reference out=w44:refnum<vi>, error out=w42:errorcluster, "Value"=w45:T3)  [unwired: 1 in]
          n32 = property class="TabCtl (strict)"(reference=w49) -> (reference out=w48:refnum<vi>, error out=w50:errorcluster, "Value"=w47:T2)  [unwired: 1 in]
          n33 = Close Reference(reference=w44, error in (no error)=w42) -> ()  [unwired: 1 out]
          n34 = Equal?(x=w45, y=T3."Begin" ("Value")) -> (x = y?=w52:bool)
          n35 = Close Reference(reference=w48, error in (no error)=w50) -> ()  [unwired: 1 out]
          n36 = Equal?(x=w47, y=T2."  Acquire  " ("Value")) -> (x = y?=w53:bool)
          n37 = And(x=w52, y=w53) -> (x .and. y?=w54:bool)
          n38 = case shown="False" w54 {
            tunnel: w40 -> [_ w77]
            frame False {
              "File Create Temp" <- TRUE ("File Create Temp")
            }
            frame True {
              n39 = local read "File Create Temp"() -> (w76:bool)
              n40 = case shown="True" w76 {
                selector: w76 -> [_ w85]
                tunnel: w77 -> [_ w86]
                frame False {
                }
                frame True {
                  n41 = Unbundle By Name(w86) -> ("Config Screen.FILE"=w87:refnum<vi>)
                  n42 = Not(x=w85) -> (.not. x?=w84:bool)
                  n43 = property class="Str"(reference=w87) -> (reference out=w89:refnum<vi>, error out=w88:errorcluster, "Value"=w79:string)  [unwired: 1 in]
                  n44 = local write "File Create Temp"(w84) -> ()
                  n45 = Close Reference(reference=w89, error in (no error)=w88) -> ()  [unwired: 1 out]
                  n46 = call "file check Unitest.vi"("file name in"=w79) -> ("file name out"=w78:string)  [unwired: 9 in, 1 out]
                  n47 = call "FILE PATH CREATION Unitest.vi"("FILE NAME :"=w78) -> ("FILE OUT"=w90:path)  [unwired: 9 in, 1 out]
                  n48 = Strip Path(path=w90) -> (name=w93:string)  [unwired: 1 out]
                  n49 = Build Path(base path=w90, name or relative path=w93) -> (appended path=w94:path)
                  n50 = Path To String(path=w94) -> (string=w91:string)
                  n51 = Concatenate Strings(w91, ".tdms" ("string")) -> (w92:string)
                  n52 = String To Path(string=w92) -> (path=w81:path)
                  n53 = TDMS Open(6:FALSE ("disable buffering (T)"), 10:T4."create or replace" ("operation"), 11:w81) -> (3:→"tdms file out":refnum<k34>)  [unwired: 4 in, 1 out]
                }
              }
            }
          }
          n54 = Unbundle By Name(w40) -> ("Motion Module.Scratch"=w68:refnum<vi>)
          n55 = local read "TDMS CLOSE"() -> (w55:bool)
          n56 = Unbundle By Name(w40) -> ("Main Screen.Trip Log"=w62:refnum<vi>)
          n57 = call "ELAPSED TIMER VI FOR MONITOR Loop.vi"("RESET"=w70, "PAUSE"=w70) -> ()  [unwired: 7 in, 3 out]
          n58 = property class="Str"(reference=w62) -> (reference out=w57:refnum<vi>, error out=w63:errorcluster, "Value"=w61:string)  [unwired: 1 in]
          n59 = case shown="True" w55 {
            selector: w55 -> [_ w74]
            frame False {
            }
            frame True {
              n60 = Not(x=w74) -> (.not. x?=w73:bool)
              n61 = local write "TDMS CLOSE"(w73) -> ()
              n62 = local read "tdms file out"() -> (w72:refnum<k34>)
              n63 = TDMS Close(11:w72) -> (0:→"error out 2":errorcluster)  [unwired: 1 in, 1 out]
            }
          }
          n64 = property class="Bool (strict)"(reference=w68) -> (reference out=w66:refnum<vi>, error out=w67:errorcluster, "Value"=w65:bool)  [unwired: 1 in]
          n65 = call "ELAPSED TIMER VI FOR MONITOR Loop for Rotary Module.vi"("RESET"=w64, "PAUSE"=w64) -> ()  [unwired: 7 in, 3 out]
          n66 = call <vilib>:"Trim Whitespace.vi"("string"=w61) -> ("trimmed string"=w60:string)  [unwired: 1 in]
          n67 = Close Reference(reference=w57, error in (no error)=w63) -> ()  [unwired: 1 out]
          n68 = String Length(string=w60) -> (length=w59:i32)
          n69 = Close Reference(reference=w66, error in (no error)=w67) -> ()  [unwired: 1 out]
          n70 = Greater Or Equal?(x=w59, y=4) -> (x >= y?=w56:bool)
          n71 = local read "Test Stop Temp"() -> (w69:bool)
          n72 = case shown="True" w69 {
            selector: w69 -> [_ w100]
            tunnel: w40 -> [_ w98]
            tunnel: w65 -> [_ w97]
            tunnel: w56 -> [_ w96]
            frame False {
            }
            frame True {
              n73 = case shown="False" w97 {
                tunnel: w98 -> [w102 _]
                tunnel: w96 -> [w101 _]
                frame False {
                  n74 = case shown="False" w101 {
                    tunnel: w102 -> [w103 _]
                    frame False {
                      n75 = call "Test Stop.vi"("Data Cluster"=w103) -> ()  [unwired: 10 in, 1 out]
                    }
                    frame True {
                    }
                  }
                }
                frame True {
                }
              }
              n76 = Not(x=w100) -> (.not. x?=w99:bool)
              n77 = local write "Test Stop Temp"(w99) -> ()
            }
          }
          n78 = call "ELAPSED TIMER VI FOR REPORT LOOP.vi"("RESET"=w41, "PAUSE"=w41) -> ()  [unwired: 7 in, 3 out]
        }
        frame True {
          w104 = 0.0  # Slip(%)
          w105 = 0.0  # ECR (ohms)
          w106 = 0.0  # MTM Disc Speed (mm/sec)
          w107 = 0.0  # MTM Ball Speed(mm/sec)
          w111 = 0.0  # Fy(N)
          w112 = 0.0  # Fx(N)
          w109 = 0.0  # MTM Disc Speed (RPM)
          w110 = 0.0  # MTM Ball Speed(RPM)
          w119 = 0.0  # Humidity ( %Rh )
          w120 = 0.0  # Mz (Nm)
          w121 = 0.0  # My (Nm)
          w122 = 0.0  # Mx (Nm)
          w118 = 0.0  # Sliding Distance (mm)
          w302 = 2.0 ("y")
          # "Rotatry Monitor Loop"
          # "Test Stop logic"
          # "Depth Monitor Loop"
          # "Friction Force  Monitor part"
          # "Load Monitor part"
          n79 = Unbundle By Name(w114) -> ("Heave AND Surge.DOWNLINK HEAVE"=w222:refnum<vi>)
          n80 = Unbundle By Name(w114) -> ("Heave AND Surge.DOWNLINK HEAVE"=w229:refnum<vi>)
          n81 = Unbundle By Name(w114) -> ("Motion Module.Rot Ver"=w242:refnum<vi>)
          n82 = case shown="True" w190 {
            tunnel: w114 -> [_ w323]
            tunnel: [FALSE ("Value") w321] -> w189
            frame False {
            }
            frame True {
              n83 = Unbundle By Name(w323) -> ("Main Screen.Scratch Start Recording"=w325:refnum<vi>)
              n84 = property class="Bool (strict)"(reference=w325) -> (reference out=w324:refnum<vi>, error out=w326:errorcluster, "Value"=w322:bool)  [unwired: 1 in]
              n85 = Not(x=w322) -> (.not. x?=w321:bool)
              n86 = Close Reference(reference=w324, error in (no error)=w326) -> ()  [unwired: 1 out]
            }
          }
          n87 = Unbundle By Name(w114) -> ("Acquostic.Downlink Packet"=w200:refnum<vi>)
          n88 = Unbundle By Name(w114) -> ("Main Screen.Set Load (N)"=w304:refnum<vi>)
          n89 = Unbundle By Name(w114) -> ("Main Screen.NL disp 2"=w314:refnum<vi>)
          n90 = Unbundle By Name(w114) -> ("Config Parameters.Heave Pulses/mm"=w296:refnum<vi>)
          n91 = Unbundle By Name(w114) -> ("Main Screen.Depthz"=w292:refnum<vi>)
          n92 = Unbundle By Name(w114) -> ("Main Screen.Test Duration"=w277:refnum<vi>)
          n93 = property class="Bool (strict)"(reference=w242) -> (reference out=w240:refnum<vi>, error out=w241:errorcluster, "Value"=w239:bool)  [unwired: 1 in]
          n94 = property class="Clust (strict)"(reference=w222) -> (reference out=w220:refnum<vi>, error out=w221:errorcluster, "Value"=w219:T5)  [unwired: 1 in]
          n95 = property on="Property Node" class="Clust (strict)"(reference=w229) -> (reference out=w231:refnum<vi>, error out=w230:errorcluster, "Value"=w228:T5)  [unwired: 1 in]
          n96 = property class="DigNum (strict)"(reference=w304) -> (reference out=w298:refnum<vi>, error out=w305:errorcluster, "Value"=w303:dbl)  [unwired: 1 in]
          n97 = property class="DigNum (strict)"(reference=w314) -> (reference out=w312:refnum<vi>, error out=w313:errorcluster, "Value"=w139:dbl)  [unwired: 1 in]
          n98 = property on="Property Node" class="Clust (strict)"(reference=w200) -> (reference out=w198:refnum<vi>, error out=w199:errorcluster, "Value"=w197:T6)  [unwired: 1 in]
          n99 = property class="Bool (strict)"(reference=w292) -> (reference out=w293:refnum<vi>, error out=w291:errorcluster, "Value"=w290:bool)  [unwired: 1 in]
          n100 = property class="DigNum (strict)"(reference=w277) -> (reference out=w278:refnum<vi>, error out=w276:errorcluster, "Value"=w275:dbl)  [unwired: 1 in]
          n101 = property class="DigNum (strict)"(reference=w296) -> (reference out=w295:refnum<vi>, error out=w297:errorcluster, "Value"=w294:dbl)  [unwired: 1 in]
          n102 = Close Reference(reference=w240, error in (no error)=w241) -> ()  [unwired: 1 out]
          n103 = Close Reference(reference=w220, error in (no error)=w221) -> ()  [unwired: 1 out]
          n104 = Unbundle By Name(w219) -> ("Spare 1"=w209:u8, "Spare 2"=w210:u8)
          n105 = Unbundle By Name(w219) -> ("Spare 3"=w202:u8, "Spare 4"=w203:u8)
          n106 = case shown="True" w239 {
            tunnel: w114 -> [_ w329]
            tunnel: [w327 w334] -> w108
            tunnel: [w327 w328] -> w149
            frame False {
              w327 = 0.0 ("Enter initial Velocity (m/s)  4")
            }
            frame True {
              n107 = Unbundle By Name(w329) -> ("Motion Module.Wear Track Diameter (mm)"=w338:refnum<vi>)
              n108 = Unbundle By Name(w329) -> ("SWAY.DOWNLINK SWAY"=w331:refnum<vi>)
              n109 = property on="Property Node" class="Clust (strict)"(reference=w331) -> (reference out=w333:refnum<vi>, error out=w332:errorcluster, "Value"=w330:T7)  [unwired: 1 in]
              n110 = property class="DigNum (strict)"(reference=w338) -> (reference out=w336:refnum<vi>, error out=w337:errorcluster, "Value"=w335:dbl)  [unwired: 1 in]
              n111 = Close Reference(reference=w333, error in (no error)=w332) -> ()  [unwired: 1 out]
              n112 = Unbundle By Name(w330) -> ("Rotary POSE"=w328:sgl)
              n113 = Close Reference(reference=w336, error in (no error)=w337) -> ()  [unwired: 1 out]
              n114 = call "rpm to mm_sec conversion.vi"("Wear Track Diameter"=w335, "Initial Speed (RPM)"=w328) -> ("Enter initial Velocity (m/s)  4"=w334:dbl)  [unwired: 7 in, 2 out]
            }
          }
          n115 = Close Reference(reference=w198, error in (no error)=w199) -> ()  [unwired: 1 out]
          n116 = Close Reference(reference=w231, error in (no error)=w230) -> ()  [unwired: 1 out]
          n117 = Unbundle By Name(w228) -> ("HEAVE POSE"=w227:sgl)
          n118 = Join Numbers(hi=w210, lo=w209) -> ((hi.lo)=w207:u16)
          n119 = Join Numbers(hi=w203, lo=w202) -> ((hi.lo)=w204:u16)
          n120 = Close Reference(reference=w298, error in (no error)=w305) -> ()  [unwired: 1 out]
          n121 = Close Reference(reference=w293, error in (no error)=w291) -> ()  [unwired: 1 out]
          n122 = Close Reference(reference=w312, error in (no error)=w313) -> ()  [unwired: 1 out]
          n123 = Type Cast(type=i16 0, x=w204) -> (*(type *) &x=w201:i16)
          n124 = Add(x=w303, y=w302) -> (x+y=w301:dbl)
          n125 = Subtract(x=w303, y=w302) -> (x-y=w300:dbl)
          n126 = Close Reference(reference=w278, error in (no error)=w276) -> ()  [unwired: 1 out]
          n127 = Unbundle By Name(w197) -> ("Signal Energy"=w123:sgl)
          n128 = Unbundle By Name(w114) -> ("Main Screen.Ambient\n Humidity"=w215:refnum<vi>)
          n129 = Close Reference(reference=w295, error in (no error)=w297) -> ()  [unwired: 1 out]
          n130 = local read "DepthZ"() -> (w288:dbl)
          n131 = Type Cast(type=i16 0, x=w207) -> (*(type *) &x=w206:i16)
          n132 = Unbundle By Name(w114) -> ("Main Screen.Main Chart 3"=w308:refnum<vi>)
          n133 = Unbundle By Name(w114) -> ("Main Screen.Ambient \nTemperature"=w218:refnum<vi>)
          n134 = Divide(x=w227, y=w294) -> (x/y=w289:dbl)
          n135 = Unbundle By Name(w114) -> ("Main Screen.NL Display 4"=w309:refnum<vi>)
          n136 = Divide(x=w201, y=u8 10) -> (x/y=w125:dbl)
          n137 = Bundle(w301, "Value"=w139, w300) -> (w299:cluster{dbl, "Value":dbl, dbl})  [unwired: 1 in]
          n138 = case shown="True" w290 {
            tunnel: w289 -> [_ w368]
            tunnel: w114 -> [_ w364]
            frame False {
            }
            frame True {
              n139 = Unbundle By Name(w364) -> ("Main Screen.Depthz"=w366:refnum<vi>)
              n140 = property class="Bool (strict)"(reference=w366, "Value"=FALSE) -> (reference out=w365:refnum<vi>, error out=w367:errorcluster)  [unwired: 1 in]
              n141 = Close Reference(reference=w365, error in (no error)=w367) -> ()  [unwired: 1 out]
              "DepthZ" <- w368
            }
          }
          n142 = Divide(x=w206, y=u8 10) -> (x/y=w124:dbl)
          n143 = property class="WFChart (strict)"(reference=w308, "Value"=w299) -> (reference out=w306:refnum<vi>, error out=w307:errorcluster)  [unwired: 1 in]
          n144 = Unbundle By Name(w114) -> ("Main Screen.Time ( HH:MM:SS ) 2"=w244:refnum<vi>)
          n145 = Unbundle By Name(w114) -> ("Main Screen.Acoustic Emission (mV)"=w195:refnum<vi>)
          n146 = property class="DigNum (strict)"(reference=w215, "Value"=w125) -> (reference out=w211:refnum<vi>, error out=w214:errorcluster)  [unwired: 1 in]
          n147 = Unbundle By Name(w114) -> ("Main Screen.gACQUOS"=w192:refnum<vi>)
          n148 = Unbundle By Name(w114) -> ("Main Screen.Depth (µm)"=w286:refnum<vi>)
          n149 = property class="DigNum (strict)"(reference=w309, "Value"=w139) -> (reference out=w311:refnum<vi>, error out=w310:errorcluster)  [unwired: 1 in]
          n150 = call "ELAPSED TIMER VI FOR MONITOR Loop.vi"("TARGET"=w275, "RESET"=FALSE ("PAUSE"), "PAUSE"=w189) -> ("ELAPSED INDICATION"=w263:bool, "ELAPSED TIMER"=w154:dbl)  [unwired: 6 in, 1 out]
          n151 = Subtract(x=w289, y=w288) -> (x-y=w281:dbl)
          n152 = property class="DigNum (strict)"(reference=w218, "Value"=w124) -> (reference out=w212:refnum<vi>, error out=w217:errorcluster)  [unwired: 1 in]
          n153 = Multiply(x=w281, y=-1000.0) -> (x*y=w150:dbl)
          n154 = Close Reference(reference=w306, error in (no error)=w307) -> ()  [unwired: 1 out]
          n155 = property class="DigNum (strict)"(reference=w244, "Value"=w154) -> (reference out=w273:refnum<vi>, error out=w274:errorcluster)  [unwired: 1 in]
          n156 = Close Reference(reference=w211, error in (no error)=w214) -> ()  [unwired: 1 out]
          n157 = Unbundle By Name(w114) -> ("Main Screen.WearGp"=w283:refnum<vi>)
          n158 = property class="WFChart (strict)"(reference=w192, "Value"=w123) -> (reference out=w193:refnum<vi>, error out=w191:errorcluster)  [unwired: 1 in]
          n159 = property class="DigNum (strict)"(reference=w286, "Value"=w150) -> (reference out=w287:refnum<vi>, error out=w285:errorcluster)  [unwired: 1 in]
          n160 = Close Reference(reference=w311, error in (no error)=w310) -> ()  [unwired: 1 out]
          n161 = property class="DigNum (strict)"(reference=w195, "Value"=w123) -> (reference out=w194:refnum<vi>, error out=w196:errorcluster)  [unwired: 1 in]
          n162 = Close Reference(reference=w212, error in (no error)=w217) -> ()  [unwired: 1 out]
          n163 = property class="WFChart (strict)"(reference=w283, "Value"=w150) -> (reference out=w284:refnum<vi>, error out=w282:errorcluster)  [unwired: 1 in]
          n164 = Unbundle By Name(w114) -> ("Main Screen.Cyclic Friction Force (N)"=w259:refnum<vi>)
          n165 = Unbundle By Name(w114) -> ("Main Screen.Friction Force (N)"=w271:refnum<vi>)
          n166 = Close Reference(reference=w273, error in (no error)=w274) -> ()  [unwired: 1 out]
          n167 = Close Reference(reference=w287, error in (no error)=w285) -> ()  [unwired: 1 out]
          n168 = Unbundle By Name(w114) -> ("Main Screen.Speed (RPM)"=w238:refnum<vi>)
          n169 = Close Reference(reference=w193, error in (no error)=w191) -> ()  [unwired: 1 out]
          n170 = Close Reference(reference=w194, error in (no error)=w196) -> ()  [unwired: 1 out]
          n171 = Close Reference(reference=w284, error in (no error)=w282) -> ()  [unwired: 1 out]
          n172 = property class="DigNum (strict)"(reference=w238, "Value"=w149) -> (reference out=w236:refnum<vi>, error out=w237:errorcluster)  [unwired: 1 in]
          n173 = property class="DigNum (strict)"(reference=w271) -> (reference out=w272:refnum<vi>, error out=w270:errorcluster, "Value"=w152:dbl)  [unwired: 1 in]
          n174 = Unbundle By Name(w114) -> ("Main Screen.Trip Log"=w233:refnum<vi>)
          n175 = call "Rotary and Traction Motor Command Send.vi"("main ref"=w114) -> ()  [unwired: 10 in, 1 out]
          n176 = property class="DigNum (strict)"(reference=w259) -> (reference out=w257:refnum<vi>, error out=w258:errorcluster, "Value"=w256:dbl)  [unwired: 1 in]
          n177 = Unbundle By Name(w114) -> ("Main Screen.Cyclic Friction Force (N) Graph"=w262:refnum<vi>)
          n178 = Unbundle By Name(w114) -> ("Motion Module.Scratch"=w243:refnum<vi>)
          n179 = Unbundle By Name(w114) -> ("Main Screen.Friction Force (N) Graph"=w245:refnum<vi>)
          n180 = property class="Str"(reference=w233) -> (reference out=w235:refnum<vi>, error out=w234:errorcluster, "Value"=w232:string)  [unwired: 1 in]
          n181 = property class="Bool (strict)"(reference=w243) -> (reference out=w251:refnum<vi>, error out=w252:errorcluster, "Value"=w250:bool)  [unwired: 1 in]
          n182 = Close Reference(reference=w236, error in (no error)=w237) -> ()  [unwired: 1 out]
          n183 = Close Reference(reference=w272, error in (no error)=w270) -> ()  [unwired: 1 out]
          n184 = Close Reference(reference=w257, error in (no error)=w258) -> ()  [unwired: 1 out]
          n185 = call <vilib>:"Trim Whitespace.vi"("string"=w232) -> ("trimmed string"=w226:string)  [unwired: 1 in]
          n186 = Unbundle By Name(w114) -> ("Main Screen.NL disp 2"=w249:refnum<vi>)
          n187 = Close Reference(reference=w235, error in (no error)=w234) -> ()  [unwired: 1 out]
          n188 = String Length(string=w226) -> (length=w225:i32)
          n189 = Unbundle By Name(w114) -> ("Main Screen.Freq (Hz)"=w147:refnum<vi>)
          n190 = Unbundle By Name(w114) -> ("Main Screen.Angle (Deg)"=w146:refnum<vi>)
          n191 = Unbundle By Name(w114) -> ("Motion Module.Wear Track Diameter (mm)"=w116:refnum<vi>)
          n192 = Unbundle By Name(w114) -> ("Motion Module.Enter Scratch Speed (mm/s):"=w130:refnum<vi>)
          n193 = Close Reference(reference=w251, error in (no error)=w252) -> ()  [unwired: 1 out]
          n194 = property class="WFChart (strict)"(reference=w262, "Value"=w256) -> (reference out=w260:refnum<vi>, error out=w261:errorcluster)  [unwired: 1 in]
          n195 = Greater Or Equal?(x=w225, y=4) -> (x >= y?=w223:bool)
          n196 = property class="WFChart (strict)"(reference=w245, "Value"=w152) -> (reference out=w268:refnum<vi>, error out=w269:errorcluster)  [unwired: 1 in]
          n197 = Unbundle By Name(w114) -> ("Main Screen.ChamberTemp"=w136:refnum<vi>)
          n198 = Unbundle By Name(w114) -> ("Main Screen.Stroke (mm)"=w133:refnum<vi>)
          n199 = property class="DigNum (strict)"(reference=w249) -> (reference out=w247:refnum<vi>, error out=w248:errorcluster, "Value"=w246:dbl)  [unwired: 1 in]
          n200 = case shown="True" w263 {
            tunnel: w114 -> [_ w342]
            tunnel: w250 -> [_ w341]
            tunnel: w223 -> [_ w340]
            frame False {
              n201 = local write "Test Stop Temp"(FALSE ("Test Stop Temp")) -> ()
            }
            frame True {
              n202 = case shown="False" w340 {
                tunnel: w342 -> [w345 _]
                tunnel: w341 -> [w344 _]
                frame False {
                  n203 = case shown="False" w344 {
                    tunnel: w345 -> [w346 _]
                    frame False {
                      (unwired) FALSE ("y")
                      n204 = Unbundle By Name(w346) -> ("Main Screen.STOP"=w352:refnum<vi>)
                      n205 = Unbundle By Name(w346) -> ("Main Screen.Start Test"=w349:refnum<vi>)
                      n206 = Unbundle By Name(w346) -> ("Main Screen.Start Test Temp"=w360:refnum<vi>)
                      n207 = Unbundle By Name(w346) -> ("Main Screen.STOP"=w359:refnum<vi>)
                      n208 = property class="Bool (strict)"(reference=w352, "Visible"=FALSE) -> (reference out=w354:refnum<vi>, error out=w353:errorcluster)  [unwired: 1 in]
                      n209 = property class="Bool (strict)"(reference=w349, "Visible"=TRUE) -> (reference out=w347:refnum<vi>, error out=w348:errorcluster)  [unwired: 1 in]
                      n210 = property class="Bool (strict)"(reference=w360, "Value"=FALSE) -> (reference out=w362:refnum<vi>, error out=w361:errorcluster)  [unwired: 1 in]
                      n211 = property class="Bool (strict)"(reference=w359, "Value"=TRUE) -> (reference out=w357:refnum<vi>, error out=w358:errorcluster)  [unwired: 1 in]
                      n212 = Close Reference(reference=w354, error in (no error)=w353) -> ()  [unwired: 1 out]
                      n213 = Close Reference(reference=w347, error in (no error)=w348) -> ()  [unwired: 1 out]
                      n214 = Close Reference(reference=w362, error in (no error)=w361) -> ()  [unwired: 1 out]
                      n215 = Close Reference(reference=w357, error in (no error)=w358) -> ()  [unwired: 1 out]
                    }
                    frame True {
                    }
                  }
                }
                frame True {
                }
              }
              "Test Stop Temp" <- TRUE ("Test Stop Temp")
            }
          }
          n216 = property class="DigNum (strict)"(reference=w147) -> (reference out=w143:refnum<vi>, error out=w148:errorcluster, "Value"=w142:dbl)  [unwired: 1 in]
          n217 = property class="DigNum (strict)"(reference=w146) -> (reference out=w144:refnum<vi>, error out=w145:errorcluster, "Value"=w141:dbl)  [unwired: 1 in]
          n218 = Close Reference(reference=w268, error in (no error)=w269) -> ()  [unwired: 1 out]
          n219 = Close Reference(reference=w260, error in (no error)=w261) -> ()  [unwired: 1 out]
          n220 = property class="DigNum (strict)"(reference=w136) -> (reference out=w135:refnum<vi>, error out=w137:errorcluster, "Value"=w128:dbl)  [unwired: 1 in]
          n221 = property class="DigNum (strict)"(reference=w133) -> (reference out=w134:refnum<vi>, error out=w132:errorcluster, "Value"=w127:dbl)  [unwired: 1 in]
          n222 = property class="DigNum (strict)"(reference=w116) -> (reference out=w115:refnum<vi>, error out=w117:errorcluster, "Value"=w113:dbl)  [unwired: 1 in]
          n223 = Unbundle By Name(w114) -> ("Main Screen.Cyclic Coefficient of Friction"=w254:refnum<vi>)
          n224 = property class="DigNum (strict)"(reference=w130) -> (reference out=w129:refnum<vi>, error out=w131:errorcluster, "Value"=w126:dbl)  [unwired: 1 in]
          n225 = Close Reference(reference=w247, error in (no error)=w248) -> ()  [unwired: 1 out]
          n226 = Unbundle By Name(w114) -> ("Main Screen.Coefficient of Friction"=w266:refnum<vi>)
          n227 = Divide(x=w256, y=w246) -> (x/y=w140:dbl)
          n228 = Close Reference(reference=w143, error in (no error)=w148) -> ()  [unwired: 1 out]
          n229 = Close Reference(reference=w144, error in (no error)=w145) -> ()  [unwired: 1 out]
          n230 = Divide(x=w152, y=w246) -> (x/y=w264:dbl)
          n231 = Close Reference(reference=w135, error in (no error)=w137) -> ()  [unwired: 1 out]
          n232 = Close Reference(reference=w134, error in (no error)=w132) -> ()  [unwired: 1 out]
          n233 = Close Reference(reference=w115, error in (no error)=w117) -> ()  [unwired: 1 out]
          n234 = Close Reference(reference=w129, error in (no error)=w131) -> ()  [unwired: 1 out]
          n235 = property class="WFChart (strict)"(reference=w266, "Value"=w264) -> (reference out=w267:refnum<vi>, error out=w265:errorcluster)  [unwired: 1 in]
          n236 = property class="WFChart (strict)"(reference=w254, "Value"=w140) -> (reference out=w253:refnum<vi>, error out=w255:errorcluster)  [unwired: 1 in]
          n237 = Close Reference(reference=w267, error in (no error)=w265) -> ()  [unwired: 1 out]
          n238 = Close Reference(reference=w253, error in (no error)=w255) -> ()  [unwired: 1 out]
          n239 = Divide(x=w140, y=w139) -> (x/y=w138:dbl)
          n240 = Divide(x=w152, y=w139) -> (x/y=w151:dbl)
          n241 = Not(x=w189) -> (.not. x?=w188:bool)
          n242 = Build Array(w139) -> (w157:dbl[])
          n243 = Build Array(w152) -> (w158:dbl[])
          n244 = Build Array(w151) -> (w159:dbl[])
          n245 = Build Array(w150) -> (w160:dbl[])
          n246 = Build Array(w149) -> (w161:dbl[])
          n247 = Build Array(w142) -> (w162:dbl[])
          n248 = Build Array(w141) -> (w163:dbl[])
          n249 = Build Array(w140) -> (w164:dbl[])
          n250 = Build Array(w138) -> (w165:dbl[])
          n251 = Build Array(w128) -> (w166:dbl[])
          n252 = Build Array(w127) -> (w167:dbl[])
          n253 = Build Array(w126) -> (w168:dbl[])
          n254 = Build Array(w125) -> (w169:dbl[])
          n255 = Build Array(w124) -> (w170:dbl[])
          n256 = Build Array(w123) -> (w171:sgl[])
          n257 = Build Array(w122) -> (w172:dbl[])
          n258 = Build Array(w121) -> (w173:dbl[])
          n259 = Build Array(w120) -> (w174:dbl[])
          n260 = Build Array(w119) -> (w175:dbl[])
          n261 = Build Array(w118) -> (w186:dbl[])
          n262 = Build Array(w113) -> (w185:dbl[])
          n263 = Build Array(w112) -> (w184:dbl[])
          n264 = Build Array(w111) -> (w183:dbl[])
          n265 = Build Array(w110) -> (w182:dbl[])
          n266 = Build Array(w109) -> (w181:dbl[])
          n267 = Build Array(w108) -> (w180:dbl[])
          n268 = Build Array(w107) -> (w179:dbl[])
          n269 = Build Array(w106) -> (w178:dbl[])
          n270 = Build Array(w105) -> (w177:dbl[])
          n271 = Build Array(w104) -> (w176:dbl[])
          n272 = Build Array(w154) -> (w153:dbl[])
          n273 = Insert Into Array(array=sgl[][] [], new element #1=w153, new element #2=w157, new element #3=w158, new element #4=w159, new element #5=w160, new element #6=w161, new element #7=w162, new element #8=w163, new element #9=w164, new element #10=w165, new element #11=w166, new element #12=w166, new element #13=w167, new element #14=w168, new element #15=w169, new element #16=w170, new element #17=w171, new element #18=w172, new element #19=w173, new element #20=w174, new element #21=w175, new element #22=w186, new element #23=w185, new element #24=w184, new element #25=w183, new element #26=w182, new element #27=w181, new element #28=w180, new element #29=w179, new element #30=w178, new element #31=w177, new element #32=w176) -> (w155:sgl[][])  [unwired: 2 in]
          n274 = case shown="True" w188 {
            tunnel: w155 -> [_ w315]
            frame False {
            }
            frame True {
              n275 = local read "tdms file out"() -> (w317:refnum<k34>)
              n276 = TDMS Write(0:w317, 5:"Measurement" ("group name in (Untitled)"), 7:string[] ["Time(Sec)", "Normal Load (N)", "Friction Force(N)", "Coefficient of Friction", " Depth (Microns)", "Speed (RPM0", "Frequency (Hz)", "Angle (Degree)", "Cyclic Friction Force (N)", "Cyclic Co-Efficient Friction Force", "Stage Temperature (Degree celcius)", "Sample Temperature (Degree celcius)", "Stroke Length (mm)", "Scratch Speed (mm/sec)", "Amb Humidity (%Rh)", "Amb Temperature (Deg C)", "Acoustic (mV)", "Mx(Nm)", "My(Nm)", "Mz (Nm)", "Humidity(%Rh)", "Sliding Distance (mm)", "Wear Track Diameter(mm)", "Fx(N)", "Fy(N)", "MTM Ball Speed(RPM)", "MTM Disc Speed (RPM)", "Entrainment Speed", "Slide Role", "Slip(%)", "Rotart Speed (m/sec)", "MTM Ball Speed (m/sec)", "MTM Disc Speed (m/sec)", "ECR (ohms)"] ("array"), 9:w315) -> (4:w316:refnum<k34>)  [unwired: 2 in, 3 out]
              n277 = local write "tdms file out"(w316) -> ()
            }
          }
          "TDMS CLOSE" <- TRUE ("TDMS CLOSE")
        }
      }
    }
    frame Error {
    }
  }
